vi "scanChartView.vi"(10 "UserEvents in":refnum<class "UserEvents.lvclass">) -> ()   [LabVIEW 2015, in "FAMTViews.lvlib"]
uses:
  FAMTViews.lvlib
  UserEvents/UserEvents.lvclass
  UserEvents/UserEvents.lvclass/UserEvents.ctl
  Typedefs/StateSelector.ctl
  Typedefs/FAMTTypedefs.lvlib
panel:
  out "Chart":cluster{dbl, dbl, dbl}(graph)
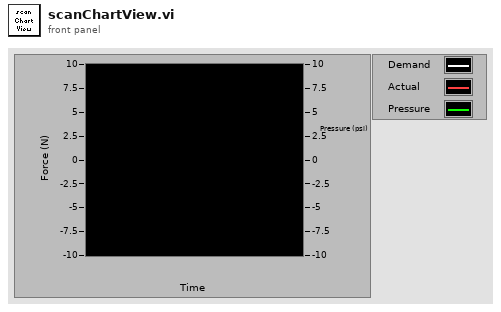
[diagram p1: front panel]
types:
  T1 = typedef "FAMTTypedefs.lvlib/PubDataEvents.ctl" = cluster{"State":refnum<user-event>, "ErrorCode":refnum<user-event>, "ADC Outputs":refnum<user-event>, "InputData":refnum<user-event>, "ControllerData":refnum<user-event>, "TestStatus":refnum<user-event>, "LogPath":refnum<user-event>, "ILC Outputs":refnum<user-event>, "Scan Progress":refnum<user-event>}
  T2 = cluster{"Event Registration Refnum":refnum<event-registration>, "Event Registration Refnum":refnum<event-registration>}
  T3 = typedef "FAMTTypedefs.lvlib/StateSelector.ctl" = enum16{"OfflineState", "FaultState", "StandbyState", "DisabledState", "EnabledState", "WaitForUserInputState", "PerformOpenLoopScanState"}
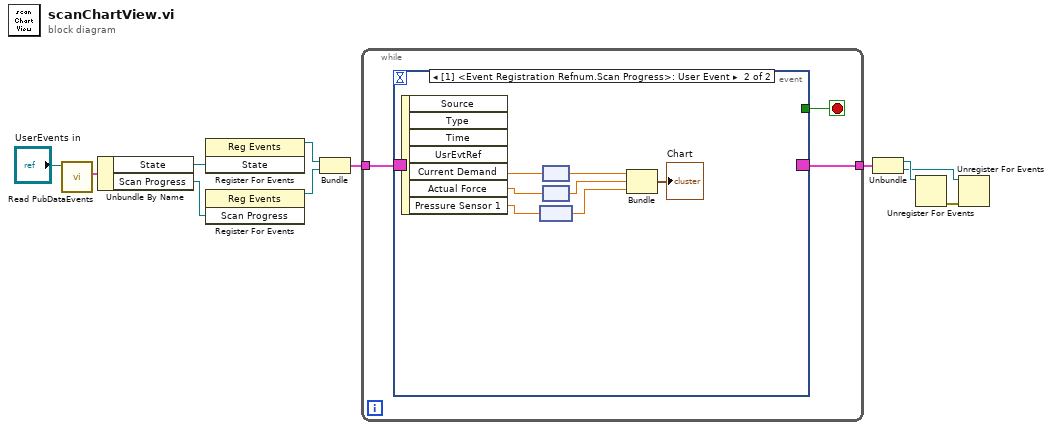
[diagram p0: block diagram]
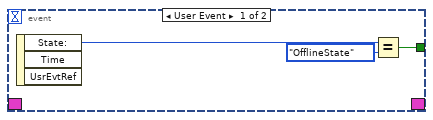
[diagram p2: hidden frame]
diagram:
  n1 = call "Read PubDataEvents.vi"("UserEvents in"="UserEvents in") -> ("PubDataEvents"=w8:T1)  [unwired: 9 in, 1 out]
  n2 = Unbundle By Name(w8) -> ("State"=w9:refnum<user-event>, "Scan Progress"=w7:refnum<user-event>)
  n3 = register-events(w9) -> (reference out=w11:refnum<event-registration>)  [unwired: 2 in, 1 out]
  n4 = register-events(w7) -> (reference out=w10:refnum<event-registration>)  [unwired: 2 in, 1 out]
  n5 = Bundle("Event Registration Refnum"=w11, "Event Registration Refnum"=w10) -> (w3:T2)  [unwired: 1 in]
  n6 = while {
    tunnel: w3 -> [w14]
    tunnel: [w13] -> w2
    stop <- w12 stop-if-true
    n7 = event shown="[1] <Event Registration Refnum.Scan Progress>: User Event" {
      selector: w14 -> [_ _]
      dyn-events: [_ _] -> w13
      timeout: _ -> [_ _]
      tunnel: [w16 _] -> w12
      event User Event {
        n8 = event-data() -> ("State:"=w15:T3)  [unwired: 1 in, 2 out]
        n9 = Equal?(x=w15, y=StateSelector."OfflineState") -> (x = y?=w16:bool)
      }
      event User Event {
        n10 = event-data() -> ("Current Demand"=w23:dbl[unit], "Actual Force"=w21:dbl[unit], "Pressure Sensor 1"=w19:dbl[unit])  [unwired: 1 in, 4 out]
        n11 = node(w19) -> (w18:dbl)
        n12 = node(w23) -> (w22:dbl)
        n13 = node(w21) -> (w20:dbl)
        n14 = Bundle(w22, w20, w18) -> (→"Chart":cluster{dbl, dbl, dbl})  [unwired: 1 in]
      }
    }
  }
  n15 = Unbundle(w2) -> ("Event Registration Refnum"=w6:refnum<event-registration>, "Event Registration Refnum"=w5:refnum<event-registration>)
  n16 = Unregister For Events(event registration refnum=w6) -> (error out=w4:errorcluster)  [unwired: 1 in]
  n17 = Unregister For Events(event registration refnum=w5, error in=w4) -> ()  [unwired: 1 out]
